vi "Probe_Channel Message.vi"(11 "Message":refnum<class "Channel Message.lvclass">) -> ()   [LabVIEW 2020, in "Channel Message.lvclass"]
doc: "This VI is used to display information about the message from a channel probe. This VI should never be used as a subVI."
uses:
  <vilib>/ChannelSupport/Channel Message/Channel Message.lvclass
  <vilib>/ChannelSupport/Channel Message/Channel Message.lvclass/Channel Message.ctl
panel:
  out "Message Class Name":string
  out "Message ID":u32
  # "To enable this probe to show detailed information about a specific message class:\n1. Open this VI:\nvi.lib\\ChannelSupport\\Channel Message\\Probe_Channel Message.vi\n2. Follow the directions on the block diagram of that VI."
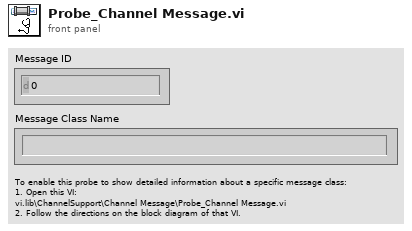
[diagram p1: front panel]
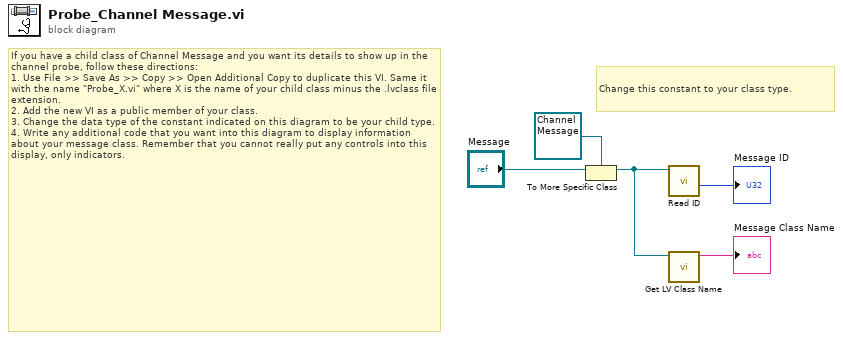
[diagram p0: block diagram]
diagram:
  # "If you have a child class of Channel Message and you want its details to show up in the channel probe, follow these directions: \n1. Use File >> Save As >> Copy >> Open Additional Copy to duplicate this VI. Same it with the name \"Probe_X.vi\" where X is the name of your child class minus the .lvclass file extension.\n2. Add the new VI as a public member of your class.\n3. Change the data type of the constant indicated on this diagram to be your child type.\n4. Write any additional code that you want into this diagram to display information about your message class. Remember that you cannot really put any controls into this display, only indicators."
  # "Change this constant to your class type."
  n1 = To More Specific Class(target class=refnum<class "Channel Message.lvclass"> refnum ("Message"), reference="Message") -> (specific class reference=w1:refnum<class "Channel Message.lvclass">)  [unwired: 1 in, 1 out]
  n2 = call <vilib>:"Read ID.vi"("Channel Message in"=w1) -> ("id"=→"Message ID":u32)  [unwired: 10 in]
  n3 = call <vilib>:"Get LV Class Name.vi"("object"=w1) -> ("class name"=→"Message Class Name":string)  [unwired: 9 in, 1 out]
